vi "Actividad 1 - LM35 y Motor.vi"() -> ()   [LabVIEW 2026]
uses:
  <vilib>/Instr/_visa.llb/VISA Configure Serial Port (Instr).vi
panel:
  out "Gauge":dbl(knob) scale=0.0..500.0
  out "Thermometer":dbl(slide) scale=0.0..100.0
  out "Contador Motor":dbl
  out "offset of match":i32
  out "match + rest of string":string
  out "substring before match":string
  in  "baud rate (9600)":u32=9600
  in  "stop":bool
  out "read buffer":string
  in  "VISA resource name":refnum<visa-resource-name>
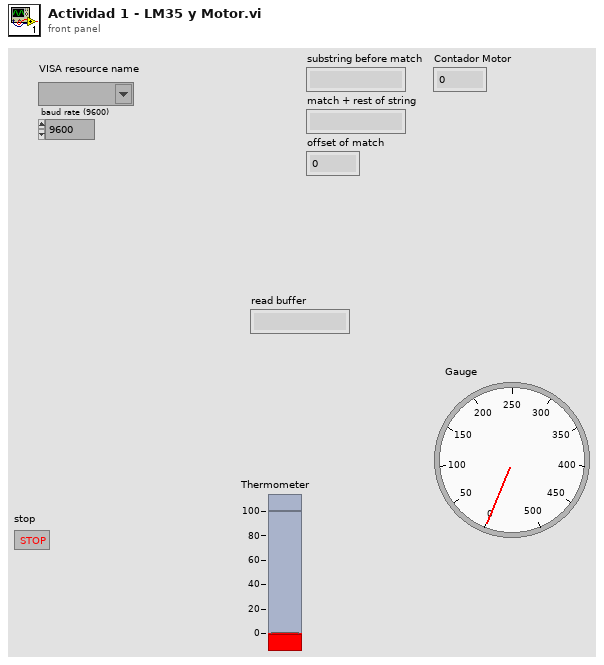
[diagram p1: front panel]
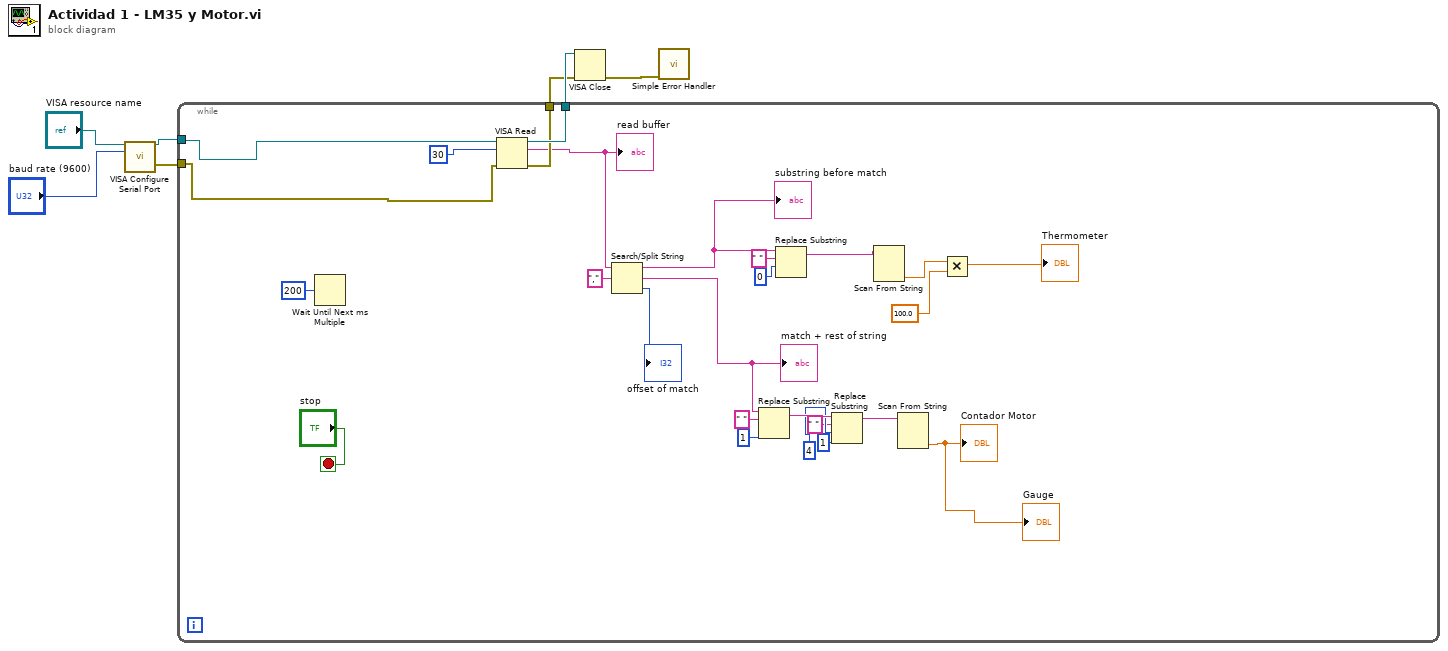
[diagram p0: block diagram]
diagram:
  n1 = call-poly "VISA Configure Serial Port"("VISA resource name"="VISA resource name", "baud rate (9600)"="baud rate (9600)") -> ("VISA resource name out"=w5:refnum<visa-resource-name>, "error out"=w4:errorcluster)  [unwired: 12 in]
  n2 = while {
    tunnel: w5 -> [w30]
    tunnel: w4 -> [w29]
    tunnel: [w28] -> w3
    tunnel: [w27] -> w2
    stop <- "stop" stop-if-true
    n3 = Wait Until Next ms Multiple(millisecond multiple=u32 200) -> ()  [unwired: 1 out]
    n4 = VISA Read(VISA resource name=w30, byte count=u32 30, error in (no error)=w29) -> (VISA resource name out=w28:refnum<visa-resource-name>, read buffer=w12:string, error out=w27:errorcluster)  [unwired: 1 out]
    "read buffer" <- w12
    n5 = Search/Split String(string=w12, search string/char (-)=",") -> (substring before match=w22:string, match + rest of string=w24:string, offset of match=→"offset of match":i32)  [unwired: 1 in]
    "substring before match" <- w22
    "match + rest of string" <- w24
    n6 = Replace Substring(2:1 ("length (len. of substring)"), 4:" " ("substring (\"\")"), 5:w24) -> (1:w25:string)  [unwired: 1 in, 1 out]
    n7 = Replace Substring(3:0 ("offset (0)"), 4:" " ("substring (\"\")"), 5:w22) -> (1:w23:string)  [unwired: 1 in, 1 out]
    n8 = Replace Substring(2:1 ("length (len. of substring)"), 3:4 ("offset (0)"), 4:" " ("substring (\"\")"), 5:w25) -> (1:w26:string)  [unwired: 1 out]
    n9 = Scan From String(input string=w23) -> (output 1=w10:dbl)  [unwired: 4 in, 3 out]
    n10 = Scan From String(input string=w26) -> (output 1=→"Contador Motor" →"Gauge":dbl)  [unwired: 4 in, 3 out]
    n11 = Multiply(x=w10, y=100.0) -> (x*y=→"Thermometer":dbl)
  }
  n12 = VISA Close(VISA resource name=w3, error in (no error)=w2) -> (error out=w1:errorcluster)
  n13 = call <vilib>:"Simple Error Handler.vi"("error in (no error)"=w1) -> ()  [unwired: 4 in, 5 out]
